vi "DefaultFromIni.vi"(8 "error in (no error)":errorcluster, 11 "AnalysisPluginsBase in":refnum<class "AnalysisPluginsBase.lvclass">) -> (0 "error out":errorcluster, 3 "AnalysisPluginsBase out":refnum<class "AnalysisPluginsBase.lvclass">)   [LabVIEW 2018, in "AnalysisPlugins.lvlib" / "AnalysisPluginsBase.lvclass"]
uses:
  AnalysisPluginsBase.lvclass
  <vilib>/Utility/config.llb/NI_LVConfig.lvlib
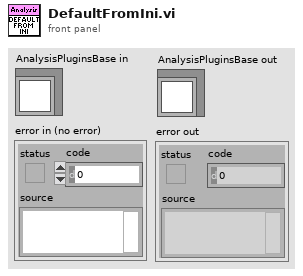
[diagram p1: front panel]
types:
  T1 = typedef "NI_LVConfig.lvlib/Config Data RefNum.ctl" = refnum<k1>
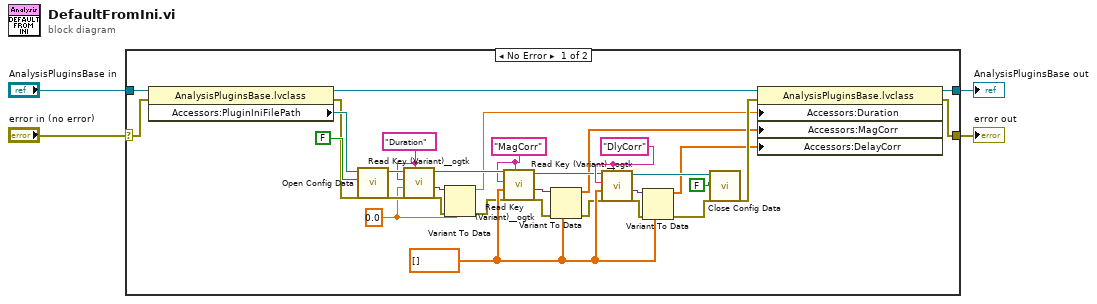
[diagram p0: block diagram]
diagram:
  n1 = case shown="No Error" "error in (no error)" {
    selector: "error in (no error)" -> [w35 w38]
    tunnel: [w7 w38] -> w3
    tunnel: [w8 w37] -> w1
    tunnel: "AnalysisPluginsBase in" -> [w36 w37]
    frame No Error {
      w26 = "DlyCorr" ("section")
      w6 = "MagCorr" ("section")
      w24 = dbl[] []
      w27 = 0.0
      w5 = "Duration" ("section")
      n2 = property class="AnalysisPluginsBase.lvclass"(reference=w36, error in=w35) -> (reference out=w13:refnum<class "AnalysisPluginsBase.lvclass">, error out=w32:errorcluster, "Accessors:PluginIniFilePath"=w34:path)
      n3 = call <vilib>:"Open Config Data.vi"("error in (no error)"=w32, "create file if necessary (T)"=FALSE, "configuration file path"=w34) -> ("error out"=w28:errorcluster, "refnum"=w29:T1)  [unwired: 6 in, 1 out]
      n4 = call <userlib>:"Read Key (Variant)__ogtk.vi"("section"=w5, "error in (no error)"=w28, "type"=w27, "key (optional)"=w5, "refnum"=w29) -> ("error out"=w30:errorcluster, "key-value"=w31:variant, "refnum out"=w17:T1)  [unwired: 3 in, 1 out]
      n5 = Variant To Data(error in=w30, type=w27, Variant=w31) -> (data=w11:dbl, error out=w18:errorcluster)
      n6 = call <userlib>:"Read Key (Variant)__ogtk.vi"("section"=w6, "error in (no error)"=w18, "type"=w24, "key (optional)"=w6, "refnum"=w17) -> ("error out"=w20:errorcluster, "key-value"=w19:variant, "refnum out"=w21:T1)  [unwired: 3 in, 1 out]
      n7 = Variant To Data(error in=w20, type=w24, Variant=w19) -> (data=w10:dbl[], error out=w22:errorcluster)
      n8 = call <userlib>:"Read Key (Variant)__ogtk.vi"("section"=w26, "error in (no error)"=w22, "type"=w24, "key (optional)"=w26, "refnum"=w21) -> ("error out"=w25:errorcluster, "key-value"=w23:variant, "refnum out"=w15:T1)  [unwired: 3 in, 1 out]
      n9 = Variant To Data(error in=w25, type=w24, Variant=w23) -> (data=w9:dbl[], error out=w16:errorcluster)
      n10 = call <vilib>:"Close Config Data.vi"("error in (no error)"=w16, "write file if changed (T)"=FALSE, "refnum"=w15) -> ("error out"=w12:errorcluster)  [unwired: 7 in, 1 out]
      n11 = property class="AnalysisPluginsBase.lvclass"(reference=w13, error in=w12, "Accessors:Duration"=w11, "Accessors:MagCorr"=w10, "Accessors:DelayCorr"=w9) -> (reference out=w8:refnum<class "AnalysisPluginsBase.lvclass">, error out=w7:errorcluster)
    }
    frame Error {
    }
  }
  "error out" <- w3
  "AnalysisPluginsBase out" <- w1
